vi "bytestream to data.vi"(9 "specifications":T1[](array[typedef]), 10 "bytestream":u8[](array[numeric]), 11 "allocation":T3) -> (3 "data table":T3)   [LabVIEW 2013, in "EIP Tags Runtime.lvclass"]
uses:
  EIP Tags Runtime.lvclass
  <vilib>/NI/Tag Bus/table/data table.ctl
  conversion specification.ctl
  <vilib>/NI/Tag Bus/tag/Data Type.ctl
  <vilib>/NI/Tag Bus/table/data polymorphs/write one/write Double.vi
  <vilib>/NI/Tag Bus/table/data polymorphs/write one/write Single.vi
  <vilib>/NI/Tag Bus/table/data polymorphs/write one/write I64.vi
  <vilib>/NI/Tag Bus/table/data polymorphs/write one/write U64.vi
  <vilib>/NI/Tag Bus/table/data polymorphs/write one/write I32.vi
  <vilib>/NI/Tag Bus/table/data polymorphs/write one/write U32.vi
  <vilib>/NI/Tag Bus/table/data polymorphs/write one/write I16.vi
  <vilib>/NI/Tag Bus/table/data polymorphs/write one/write U16.vi
  <vilib>/NI/Tag Bus/table/data polymorphs/write one/write I8.vi
  <vilib>/NI/Tag Bus/table/data polymorphs/write one/write U8.vi
  <vilib>/NI/Tag Bus/table/data polymorphs/write one/write Boolean.vi
  <vilib>/NI/Tag Bus/table/data table.lvlib
  <vilib>/NI/Tag Bus/tag/tag descriptor.lvclass
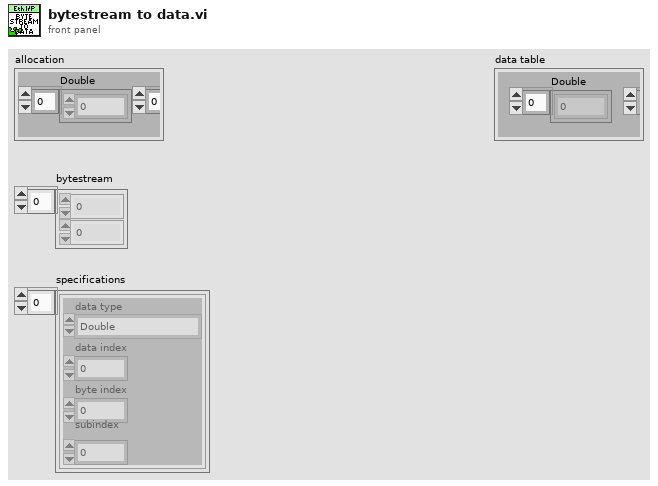
[diagram p1: front panel]
types:
  T1 = typedef "EIP Tags Runtime.lvclass/conversion specification.ctl" = cluster{"data type":T2, "data index":i32, "byte index":i32, "subindex":i32}
  T2 = typedef "tag bus.lvlib/tag descriptor.lvclass/Data Type.ctl" = enum16{"Double", "Single", "I64", "I32", "I16", "I8", "U64", "U32", "U16", "U8", "Boolean", "String", "Array of Double", "Array of Single", "Array of I64", "Array of I32", "Array of I16", "Array of I8", "Array of U64", "Array of U32", "Array of U16", "Array of U8", "Array of Boolean", "Array of String"}
  T3 = typedef "tag bus.lvlib/data table.lvlib/data table.ctl" = cluster{"Double":dbl[], "Single":sgl[], "I64":i64[], "I32":i32[], "I16":i16[], "I8":i8[], "U64":u64[], "U32":u32[], "U16":u16[], "U8":u8[], "Boolean":bool[], "String":string[], "Array of Double":cluster{"DBL Array":dbl[]}[], "Array of Single":cluster{"SGL Array":sgl[]}[], "Array of I64":cluster{"I64 Array":i64[]}[], "Array of I32":cluster{"I32 Array":i32[]}[], "Array of I16":cluster{"I16 Array":i16[]}[], "Array of I8":cluster{"I8 Array":i8[]}[], "Array of U64":cluster{"U64 Array":u64[]}[], "Array of U32":cluster{"U32 Array":u32[]}[], "Array of U16":cluster{"U16 Array":u16[]}[], "Array of U8":cluster{"U8 Array":u8[]}[], "Array of Boolean":cluster{"Boolean Array":bool[]}[], "Array of String":cluster{"String Array":string[]}[]}
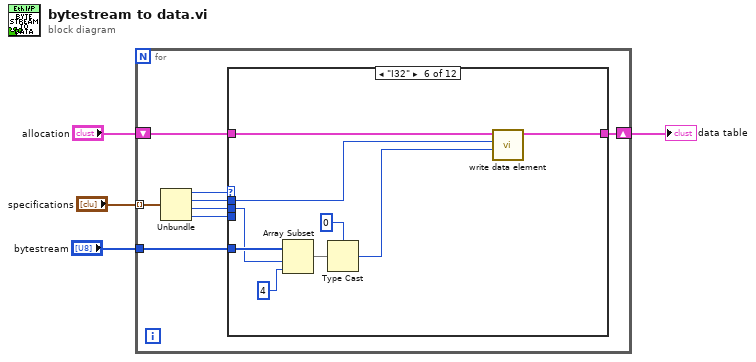
[diagram p0: block diagram]
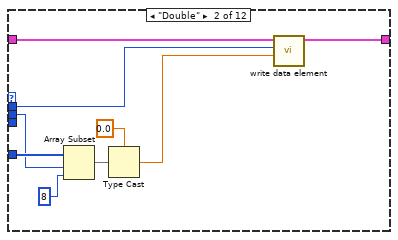
[diagram p3: hidden frame]
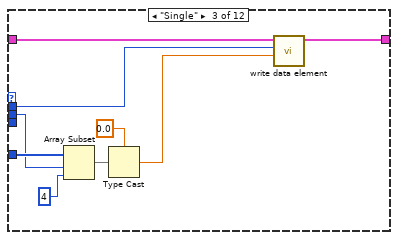
[diagram p4: hidden frame]
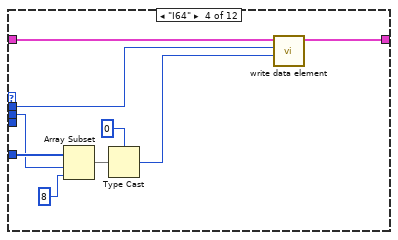
[diagram p5: hidden frame]
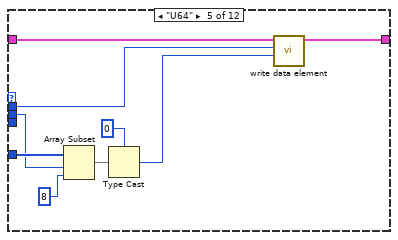
[diagram p6: hidden frame]
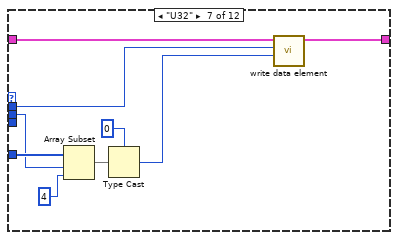
[diagram p7: hidden frame]
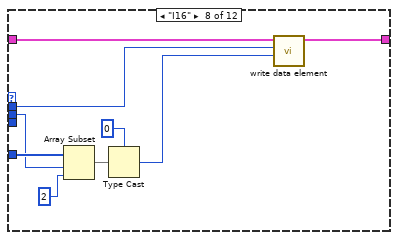
[diagram p8: hidden frame]
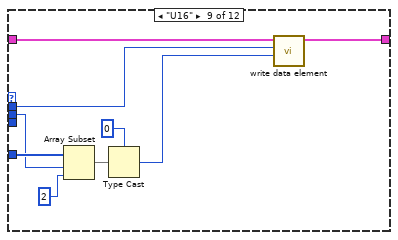
[diagram p9: hidden frame]
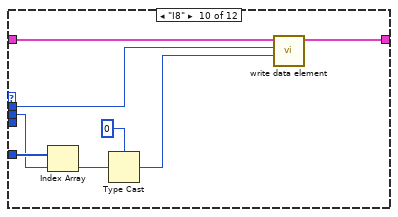
[diagram p10: hidden frame]
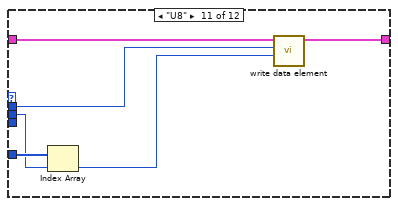
[diagram p11: hidden frame]
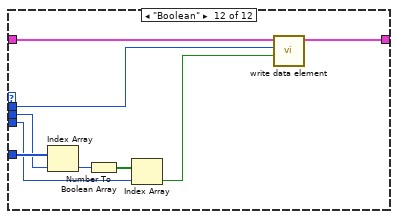
[diagram p12: hidden frame]
diagram:
  n1 = for {
    shift-right: [w9] -> w3
    shift-left: "allocation" -> [w10]
    tunnel: "bytestream" -> [w8]
    tunnel: "specifications" -> [w12] mode=indexing
    n2 = Unbundle(w12) -> ("data type"=w11:T2, "data index"=w7:i32, "byte index"=w5:i32, "subindex"=w6:i32)
    n3 = case shown="\"I32\"" w11 {
      tunnel: w10 -> [w13 w22 w31 w40 w49 w58 w67 w76 w85 w93 w99 w108]
      tunnel: [w13 w21 w30 w39 w48 w57 w66 w75 w84 w92 w98 w107] -> w9
      tunnel: w5 -> [_ w18 w27 w36 w45 w54 w63 w72 w81 w90 w96 w105]
      tunnel: w8 -> [_ w20 w29 w38 w47 w56 w65 w74 w83 w91 w97 w106]
      tunnel: w7 -> [_ w17 w26 w35 w44 w53 w62 w71 w80 w89 w95 w104]
      tunnel: w6 -> [_ _ _ _ _ _ _ _ _ _ _ w100]
      frame Default {
      }
      frame "Double" {
        n4 = Array Subset(array=w20, index=w18, length=8 ("x")) -> (w16:u8[])
        n5 = Type Cast(type=0.0, x=w16) -> (*(type *) &x=w14:dbl)
        n6 = call-poly <vilib>:"write data element.vi"("value"=w14, "index"=w17, "data table in"=w22) -> ("data table out"=w21:T3)  [unwired: 8 in]
      }
      frame "Single" {
        n7 = Array Subset(array=w29, index=w27, length=4 ("x")) -> (w25:u8[])
        n8 = Type Cast(type=sgl 0.0, x=w25) -> (*(type *) &x=w23:sgl)
        n9 = call-poly <vilib>:"write data element.vi"("value"=w23, "index"=w26, "data table in"=w31) -> ("data table out"=w30:T3)  [unwired: 8 in]
      }
      frame "I64" {
        n10 = Array Subset(array=w38, index=w36, length=8 ("x")) -> (w34:u8[])
        n11 = Type Cast(type=i64 0, x=w34) -> (*(type *) &x=w32:i64)
        n12 = call-poly <vilib>:"write data element.vi"("value"=w32, "index"=w35, "data table in"=w40) -> ("data table out"=w39:T3)  [unwired: 8 in]
      }
      frame "U64" {
        n13 = Array Subset(array=w47, index=w45, length=8 ("x")) -> (w43:u8[])
        n14 = Type Cast(type=u64 0, x=w43) -> (*(type *) &x=w41:u64)
        n15 = call-poly <vilib>:"write data element.vi"("value"=w41, "index"=w44, "data table in"=w49) -> ("data table out"=w48:T3)  [unwired: 8 in]
      }
      frame "I32" {
        n16 = Array Subset(array=w56, index=w54, length=4 ("x")) -> (w52:u8[])
        n17 = Type Cast(type=0, x=w52) -> (*(type *) &x=w50:i32)
        n18 = call-poly <vilib>:"write data element.vi"("value"=w50, "index"=w53, "data table in"=w58) -> ("data table out"=w57:T3)  [unwired: 8 in]
      }
      frame "U32" {
        n19 = Array Subset(array=w65, index=w63, length=4 ("x")) -> (w61:u8[])
        n20 = Type Cast(type=u32 0, x=w61) -> (*(type *) &x=w59:u32)
        n21 = call-poly <vilib>:"write data element.vi"("value"=w59, "index"=w62, "data table in"=w67) -> ("data table out"=w66:T3)  [unwired: 8 in]
      }
      frame "I16" {
        n22 = Array Subset(array=w74, index=w72, length=2 ("x")) -> (w70:u8[])
        n23 = Type Cast(type=i16 0, x=w70) -> (*(type *) &x=w68:i16)
        n24 = call-poly <vilib>:"write data element.vi"("value"=w68, "index"=w71, "data table in"=w76) -> ("data table out"=w75:T3)  [unwired: 8 in]
      }
      frame "U16" {
        n25 = Array Subset(array=w83, index=w81, length=2 ("x")) -> (w79:u8[])
        n26 = Type Cast(type=u16 0, x=w79) -> (*(type *) &x=w77:u16)
        n27 = call-poly <vilib>:"write data element.vi"("value"=w77, "index"=w80, "data table in"=w85) -> ("data table out"=w84:T3)  [unwired: 8 in]
      }
      frame "I8" {
        n28 = Index Array(array=w91, index=w90) -> (element=w88:u8)
        n29 = Type Cast(type=i8 0, x=w88) -> (*(type *) &x=w86:i8)
        n30 = call-poly <vilib>:"write data element.vi"("value"=w86, "index"=w89, "data table in"=w93) -> ("data table out"=w92:T3)  [unwired: 8 in]
      }
      frame "U8" {
        n31 = Index Array(array=w97, index=w96) -> (element=w94:u8)
        n32 = call-poly <vilib>:"write data element.vi"("value"=w94, "index"=w95, "data table in"=w99) -> ("data table out"=w98:T3)  [unwired: 8 in]
      }
      frame "Boolean" {
        n33 = Index Array(array=w106, index=w105) -> (element=w103:u8)
        n34 = Number To Boolean Array(number=w103) -> (Boolean array=w102:bool[])
        n35 = Index Array(array=w102, index=w100) -> (element=w101:bool)
        n36 = call-poly <vilib>:"write data element.vi"("value"=w101, "index"=w104, "data table in"=w108) -> ("data table out"=w107:T3)  [unwired: 8 in]
      }
    }
  }
  "data table" <- w3
